vi "Parse Status.vi"(1 "Buffer in":string) -> (0 "status":string)   [LabVIEW 2019, in "PGC2D.lvlib"]
uses:
  PGC2D.lvlib
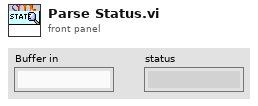
[diagram p1: front panel]
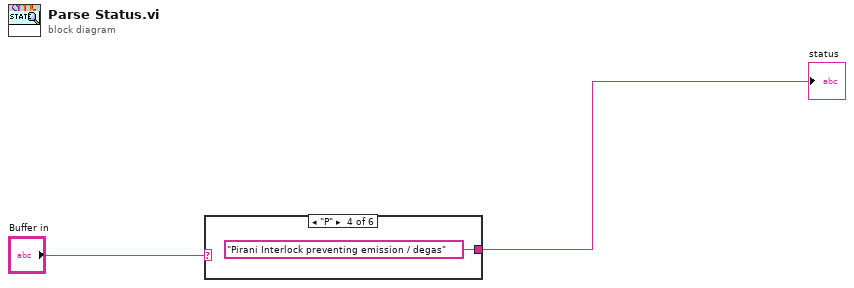
[diagram p0: block diagram]
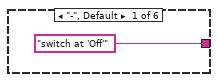
[diagram p2: hidden frame]
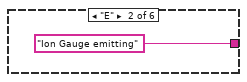
[diagram p3: hidden frame]
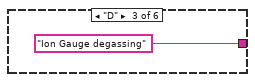
[diagram p4: hidden frame]
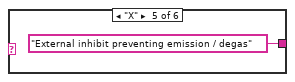
[diagram p5: hidden frame]
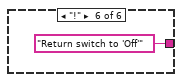
[diagram p6: hidden frame]
diagram:
  n1 = case shown="\"P\"" "Buffer in" {
    tunnel: ["switch at 'Off'" ("replace string (\"\")") "Ion Gauge emitting" ("replace string (\"\")") "Ion Gauge degassing" ("replace string (\"\")") "Pirani Interlock preventing emission / degas" ("replace string (\"\")") "External inhibit preventing emission / degas" ("replace string (\"\")") "Return switch to 'Off'" ("replace string (\"\")")] -> w2
    frame "-", Default {
    }
    frame "E" {
    }
    frame "D" {
    }
    frame "P" {
    }
    frame "X" {
    }
    frame "!" {
    }
  }
  "status" <- w2
